vi "OutputSwerve.vi"() -> ()   [LabVIEW 2020]
doc: "This VI runs feedback and feedforward controllers, manages safety interlocks, and sends commands to the swerve drive and azimuth motors. This VI also controls the commanded drive shifter (low gear or high gear) state."
uses:
  744fb9e7-64fc-4bc7-b371-cd49665d8c00.vi
  bd7bff45-d105-4c72-b52f-b7d898b15bf8.vi
  e7293d0b-e8ab-4975-ac5b-493dfa430016.vi
  4db519e9-bae7-49f3-a1c3-53a7204bbb79.vi
  d610c66c-71b6-4d3a-a8b1-b399ee96c8a2.vi
  77f8b8d5-fd7b-4b62-a195-6ccd341d14a1.vi
  6abf8b40-ef0a-49e3-8d46-47362e9bd307.vi
  ae5b7493-7bbf-44c5-8d67-5f44d96a3e48.vi
  GlobalDriverStationData.vi
  GlobalDrivebase.vi
  TAI_Motor.vi
  GRNF_CTREMotor.vi
  GRNF_GenericSolenoid.vi
  TAI_Solenoid.vi
panel:
  in  "Azimuth PID Parameters":T1={"Kp"=0.3, "Ki"=0.0, "Kd"=0.0, "Kf (don't use)"=0.0, "I-Zone"=10.0} {"Kd" min=0.0; "Ki" min=0.0; "Kp" min=0.0}
  in  "Manual Azimuth Goal (deg) [-180,180]":dbl step=5.0
  in  "Manually Override Azimuth Goal":bool
  in  "Best Angle Hysteresis (deg)":dbl=20.0 format="%#_13g"
  out "Azimuth Position":cluster{dbl, "Interlock Output":dbl}(graph)
  out "Azimuth Error (deg)":dbl
  in  "Plotting":T2(ring)
  in  "Force to Low Gear":bool
  in  "Force To High Gear":bool
  in  "Drive Command Override [0,1]":dbl min=0.0 max=1.0 step=0.1
  in  "Manually Override Drive Command":bool
  in  "Time Below Speed (ms)":u32=150
  in  "Time Above Speed (ms)":u32=150
  in  "Switch to Low Gear (rpm)":dbl=500.0
  in  "Switch to High Gear (rpm)":dbl=3500.0
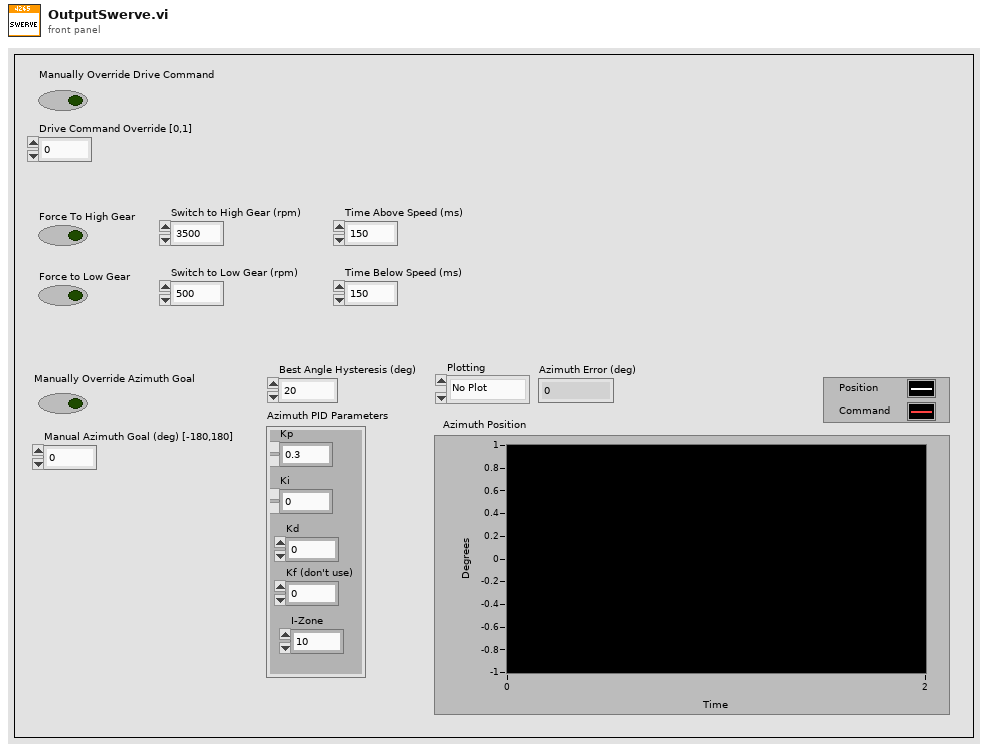
[diagram p1: front panel]
types:
  T1 = cluster{"Kp":dbl, "Ki":dbl, "Kd":dbl, "Kf (don't use)":dbl, "I-Zone":dbl}
  T2 = enum16{"No Plot", "Module 0", "Module 1", "Module 2", "Module 3"}
  T3 = enum16{"Safety", "Travelling", "Positioning", "Holding"}
  T4 = typedef "WPI_MotorControlDeviceRef.ctl" = cluster{"DeviceStatus":errorcluster, "Type":T5, "PWM":cluster{"PWM Channel":T6, "DeadBand":T7}, "CAN":cluster{"Device Number":u8, "SetOutput VI Ref":variant, "GetOutput VI Ref":variant, "Enable VI Ref":variant, "Disable VI Ref":variant, "Data":variant}, "Invert":bool, "DIO PWM":cluster{"PWM \"Enable\" Channel":T6, "DIOChannel":T8, "PWM Rate":dbl}}
  T5 = typedef "WPI_MotorControlType.ctl" = enum16{"PWM", "CAN", "DIO PWM"}
  T6 = typedef "FPGA_DIOPWMChannel.ctl" = enum8{"PWM 0", "PWM 1", "PWM 2", "PWM 3", "PWM 4", "PWM 5", "PWM 6", "PWM 7", "PWM 8", "PWM 9", "PWM MXP 0", "PWM MXP 1", "PWM MXP 2", "PWM MXP 3", "PWM MXP 4", "PWM MXP 5", "PWM MXP 6", "PWM MXP 7", "PWM MXP 8", "PWM MXP 9", "Invalid"}
  T7 = typedef "WPI_PWMDeadband.ctl" = cluster{"Name":string, "maxPositivePwm":i32, "minPositivePwm":i32, "centerPwm":i32, "maxNegativePwm":i32, "minNegativePwm":i32, "angularRange":u16}
  T8 = typedef "FPGA_DIOChannel.ctl" = enum8{"DIO 0", "DIO 1", "DIO 2", "DIO 3", "DIO 4", "DIO 5", "DIO 6", "DIO 7", "DIO 8", "DIO 9", "DIO MXP 0", "DIO MXP 1", "DIO MXP 2", "DIO MXP 3", "DIO MXP 4", "DIO MXP 5", "DIO MXP 6", "DIO MXP 7", "DIO MXP 8", "DIO MXP 9", "DIO MXP 10", "DIO MXP 11", "DIO MXP 12", "DIO MXP 13", "DIO MXP 14", "DIO MXP 15", "SPI Port CS1", "SPI Port CS2", "SPI Port CS3", "SPI Port MISO", "SPI Port MOSI", "Invalid"}
  T9 = enum16{"No Changed Output", "New Normal Output", "New Testing Output"}
  T10 = enum16{"Low Gear", "High Gear", "Transiting", "Unknown", "Force Low Gear"}
  T11 = cluster{"SEN_Azimuth_Position_Unwrapped_3 (deg)":dbl, dbl}
  T12 = typedef "WPI_SolenoidDevRef.ctl" = cluster{"DevStatus":errorcluster, "Pneumatics Control Module":u8, "Forward Solenoid Channel":T13, "Reverse Solenoid Channel":T13}
  T13 = typedef "WPI_SolenoidChannel.ctl" = enum8{"Solenoid 0", "Solenoid 1", "Solenoid 2", "Solenoid 3", "Solenoid 4", "Solenoid 5", "Solenoid 6", "Solenoid 7", "Solenoid 8", "Solenoid 9", "Solenoid 10", "Solenoid 11", "Solenoid 12", "Solenoid 13", "Solenoid 14", "Solenoid 15", "Invalid"}
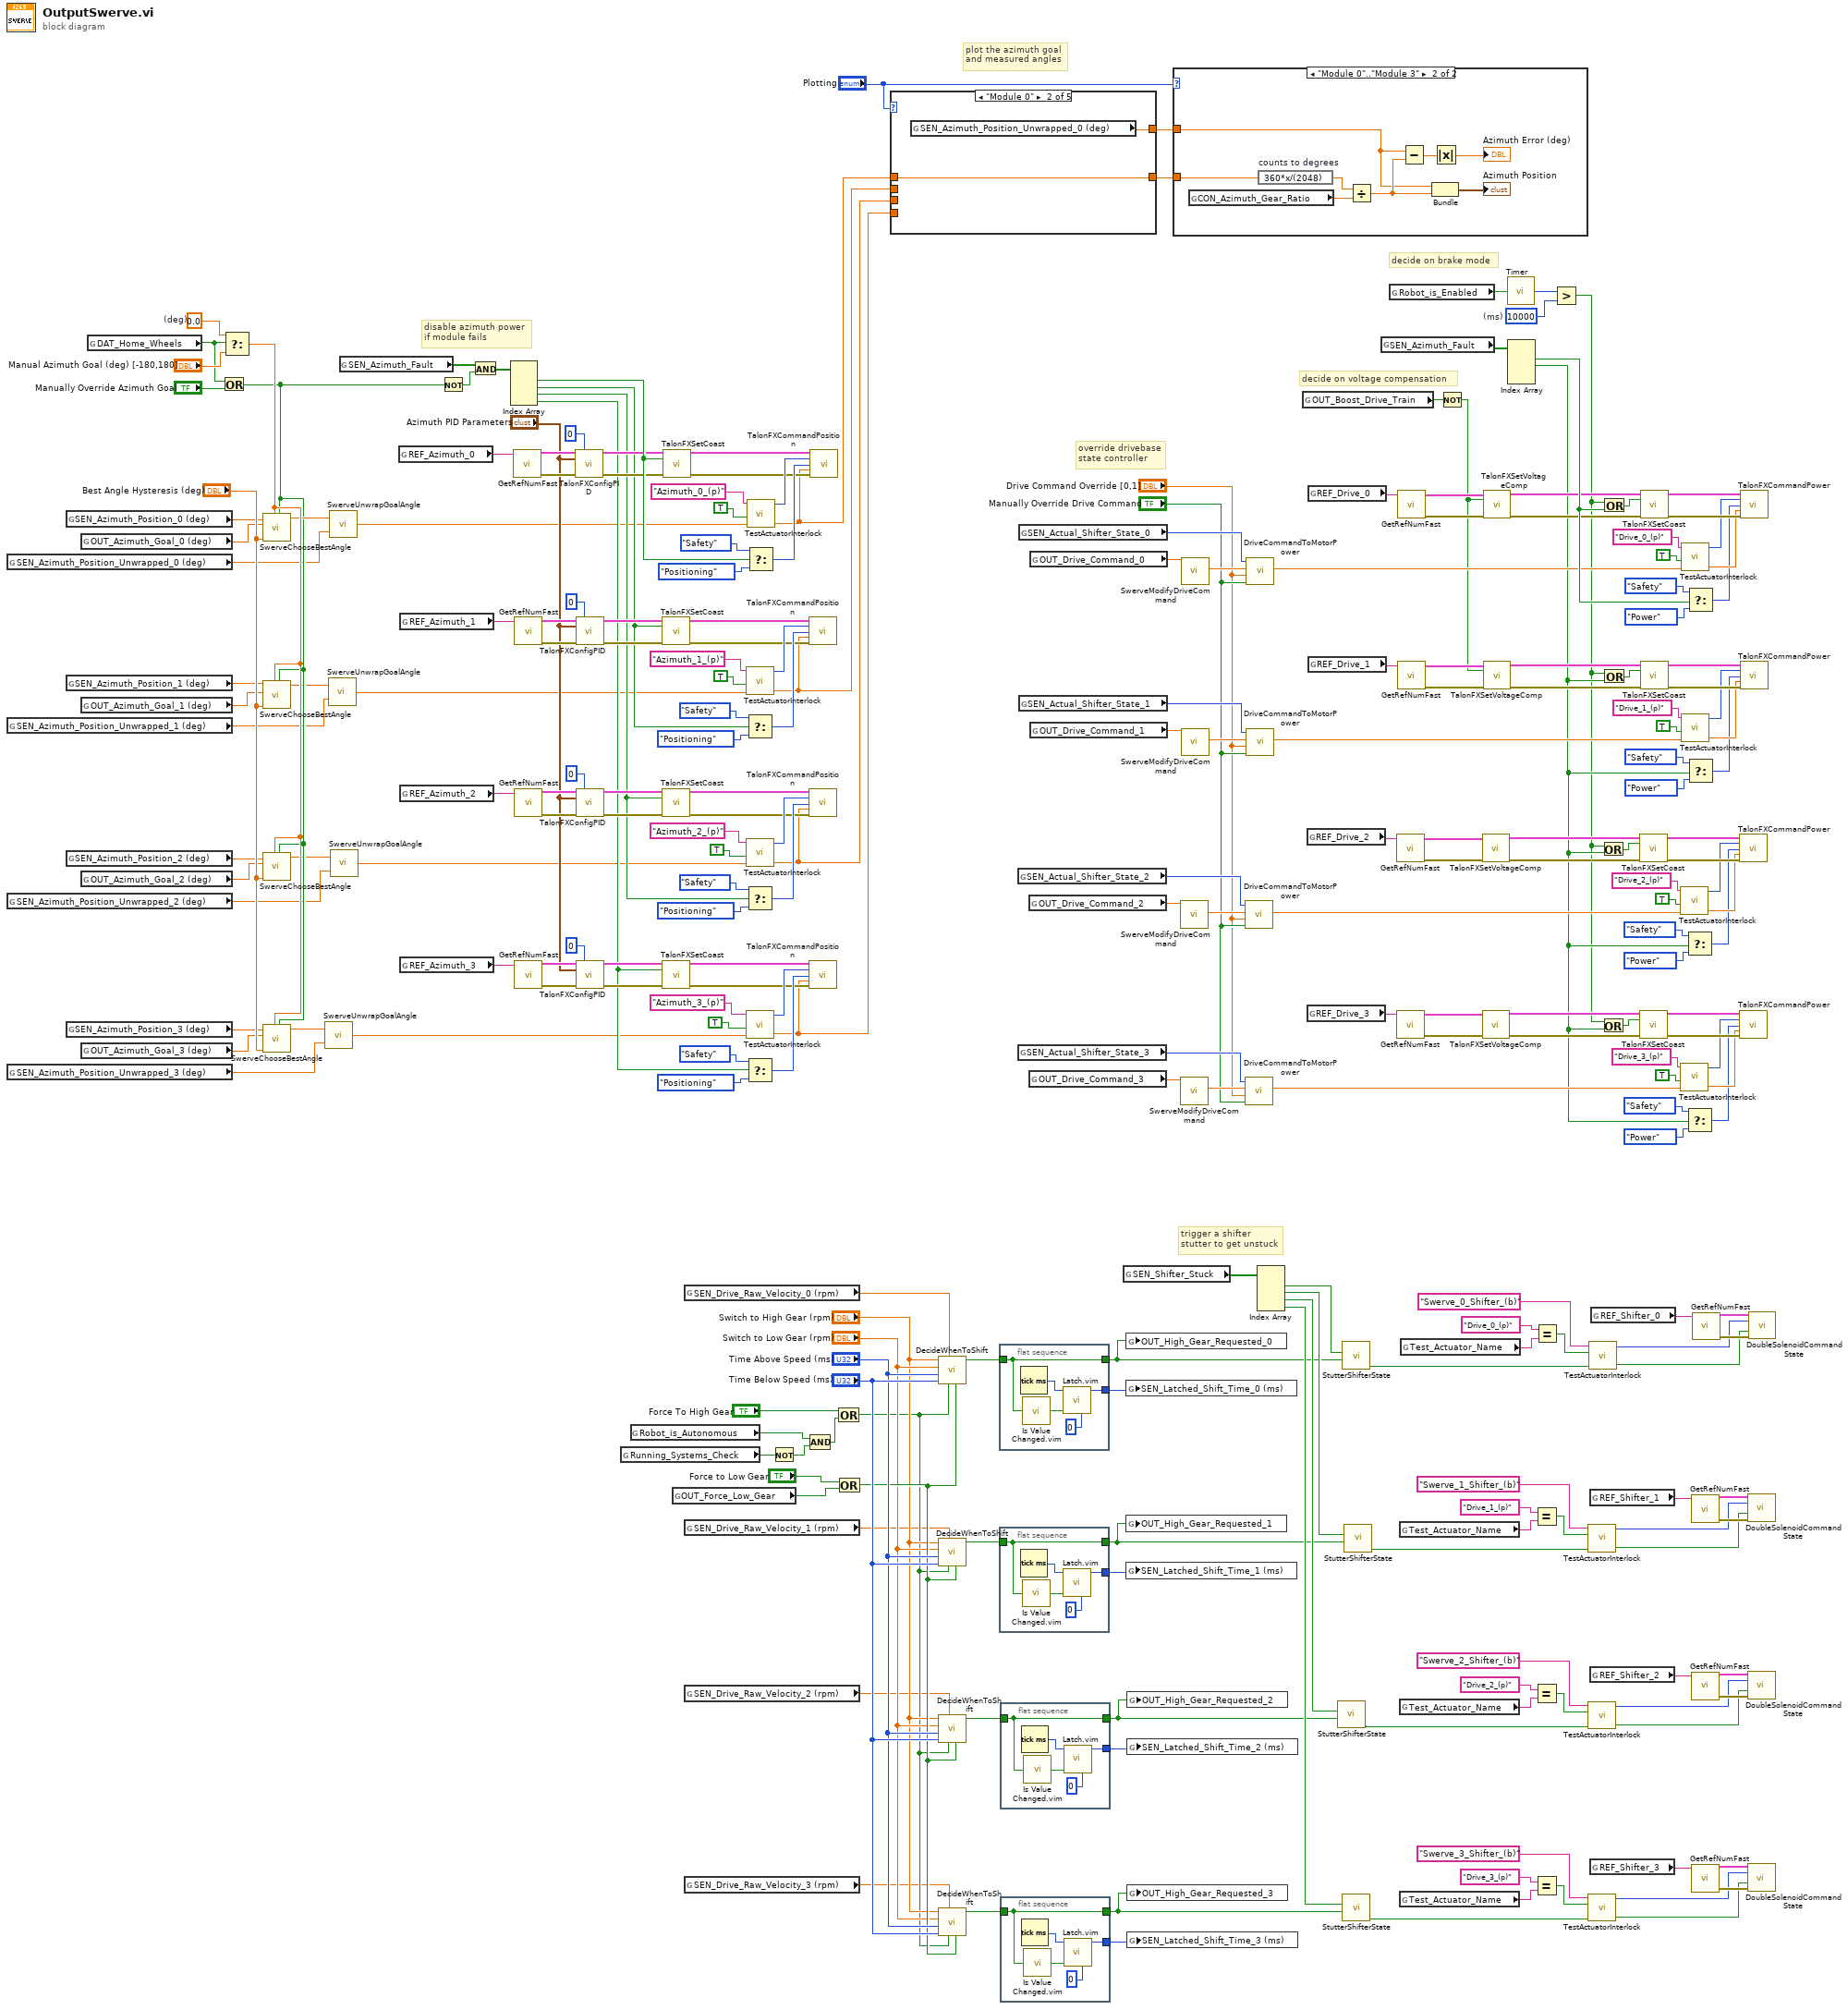
[diagram p0: block diagram]
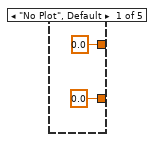
[diagram p3: hidden frame]
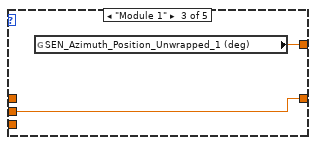
[diagram p4: hidden frame]
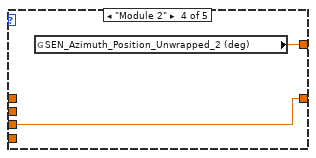
[diagram p5: hidden frame]
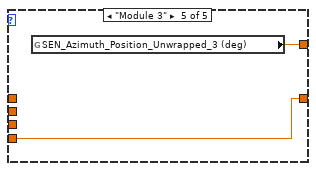
[diagram p6: hidden frame]
diagram:
  w97 = 0.0  # (deg)
  w230 = u32 10000  # (ms)
  # "plot the azimuth goal\nand measured angles"
  # "disable azimuth power\nif module fails"
  # "trigger a shifter\nstutter to get unstuck"
  # "override drivebase\nstate controller"
  # "decide on brake mode"
  # "decide on voltage compensation"
  n1 = global read "GlobalDrivebase.vi" "SEN_Azimuth_Position_Unwrapped_0 (deg)"() -> (w80:dbl)
  n2 = global read "GlobalDrivebase.vi" "SEN_Azimuth_Position_Unwrapped_1 (deg)"() -> (w78:dbl)
  n3 = global read "GlobalDrivebase.vi" "SEN_Azimuth_Position_Unwrapped_2 (deg)"() -> (w76:dbl)
  n4 = global read "GlobalDrivebase.vi" "SEN_Azimuth_Position_Unwrapped_3 (deg)"() -> (w74:dbl)
  n5 = global read "GlobalDrivebase.vi" "SEN_Azimuth_Position_0 (deg)"() -> (w81:dbl)
  n6 = global read "GlobalDrivebase.vi" "SEN_Azimuth_Position_1 (deg)"() -> (w79:dbl)
  n7 = global read "GlobalDrivebase.vi" "SEN_Azimuth_Position_2 (deg)"() -> (w77:dbl)
  n8 = global read "GlobalDrivebase.vi" "SEN_Azimuth_Position_3 (deg)"() -> (w75:dbl)
  n9 = global read "GlobalDrivebase.vi" "OUT_Azimuth_Goal_0 (deg)"() -> (w85:dbl)
  n10 = global read "GlobalDrivebase.vi" "OUT_Azimuth_Goal_1 (deg)"() -> (w84:dbl)
  n11 = global read "GlobalDrivebase.vi" "OUT_Azimuth_Goal_2 (deg)"() -> (w83:dbl)
  n12 = global read "GlobalDrivebase.vi" "OUT_Azimuth_Goal_3 (deg)"() -> (w82:dbl)
  n13 = global read "GlobalDrivebase.vi" "DAT_Home_Wheels"() -> (w10:bool)
  n14 = Or(x=w10, y="Manually Override Azimuth Goal") -> (x .or. y?=w90:bool)
  n15 = Select(t=w97, s=w10, f="Manual Azimuth Goal (deg) [-180,180]") -> (s? t:f=w96:dbl)
  n16 = call "SwerveChooseBestAngle.vi"("Goal Override"=w90, "Goal Override Angle (deg) [-180,+180]"=w96, "Hysteresis (deg)"="Best Angle Hysteresis (deg)", "Goal Angle (deg) [-180,+180]"=w85, "Current Angle (deg) [-180,+180]"=w81) -> ("Flipped Goal Angle (deg) [-180, +180]"=w94:dbl)  [unwired: 4 in, 2 out]
  n17 = call "SwerveChooseBestAngle.vi"("Goal Override"=w90, "Goal Override Angle (deg) [-180,+180]"=w96, "Hysteresis (deg)"="Best Angle Hysteresis (deg)", "Goal Angle (deg) [-180,+180]"=w84, "Current Angle (deg) [-180,+180]"=w79) -> ("Flipped Goal Angle (deg) [-180, +180]"=w88:dbl)  [unwired: 4 in, 2 out]
  n18 = call "SwerveChooseBestAngle.vi"("Goal Override"=w90, "Goal Override Angle (deg) [-180,+180]"=w96, "Hysteresis (deg)"="Best Angle Hysteresis (deg)", "Goal Angle (deg) [-180,+180]"=w83, "Current Angle (deg) [-180,+180]"=w77) -> ("Flipped Goal Angle (deg) [-180, +180]"=w87:dbl)  [unwired: 4 in, 2 out]
  n19 = call "SwerveChooseBestAngle.vi"("Goal Override"=w90, "Goal Override Angle (deg) [-180,+180]"=w96, "Hysteresis (deg)"="Best Angle Hysteresis (deg)", "Goal Angle (deg) [-180,+180]"=w82, "Current Angle (deg) [-180,+180]"=w75) -> ("Flipped Goal Angle (deg) [-180, +180]"=w86:dbl)  [unwired: 4 in, 2 out]
  n20 = call "SwerveUnwrapGoalAngle.vi"("Current Unwrapped Angle (deg) [-Inf,+Inf]"=w74, "Flipped Goal Angle (deg) [-180, +180]"=w86) -> ("Absolute Azimuth Position (tics) [-Inf,+Inf]"=w11:dbl)
  n21 = call "SwerveUnwrapGoalAngle.vi"("Current Unwrapped Angle (deg) [-Inf,+Inf]"=w78, "Flipped Goal Angle (deg) [-180, +180]"=w88) -> ("Absolute Azimuth Position (tics) [-Inf,+Inf]"=w13:dbl)
  n22 = call "SwerveUnwrapGoalAngle.vi"("Current Unwrapped Angle (deg) [-Inf,+Inf]"=w80, "Flipped Goal Angle (deg) [-180, +180]"=w94) -> ("Absolute Azimuth Position (tics) [-Inf,+Inf]"=w14:dbl)
  n23 = call "SwerveUnwrapGoalAngle.vi"("Current Unwrapped Angle (deg) [-Inf,+Inf]"=w76, "Flipped Goal Angle (deg) [-180, +180]"=w87) -> ("Absolute Azimuth Position (tics) [-Inf,+Inf]"=w12:dbl)
  n24 = global read "GlobalDrivebase.vi" "SEN_Azimuth_Fault"() -> (w73:bool[])
  n25 = global read "GlobalDrivebase.vi" "REF_Azimuth_0"() -> (w98:string)
  n26 = global read "GlobalDrivebase.vi" "REF_Azimuth_1"() -> (w59:string)
  n27 = global read "GlobalDrivebase.vi" "REF_Azimuth_2"() -> (w45:string)
  n28 = global read "GlobalDrivebase.vi" "REF_Azimuth_3"() -> (w29:string)
  n29 = Not(x=w90) -> (.not. x?=w91:bool)
  n30 = And(x=w73, y=w91) -> (x .and. y?=w92:bool[])
  n31 = Index Array(array=w92) -> (element #1=w66:bool, element #2=w47:bool, element #3=w33:bool, element #4=w15:bool)  [unwired: 4 in]
  n32 = call-poly "GetRefNumFast.vi"("RefNum Name"=w98) -> ("Error"=w62:errorcluster, "Device Reference"=w61:T4)  [unwired: 5 in]
  n33 = call-poly "GetRefNumFast.vi"("RefNum Name"=w59) -> ("Error"=w50:errorcluster, "Device Reference"=w49:T4)  [unwired: 5 in]
  n34 = call-poly "GetRefNumFast.vi"("RefNum Name"=w45) -> ("Error"=w36:errorcluster, "Device Reference"=w35:T4)  [unwired: 5 in]
  n35 = call-poly "GetRefNumFast.vi"("RefNum Name"=w29) -> ("Error"=w20:errorcluster, "Device Reference"=w19:T4)  [unwired: 5 in]
  n36 = call "TalonFXConfigPID.vi"("Device Reference (in)"=w61, "PID Slot"=0 ("slotIdx"), "PID Parameters"="Azimuth PID Parameters", "Error (in)"=w62) -> ("Device Reference (out)"=w64:T4, "Error (out)"=w63:errorcluster)  [unwired: 10 in]
  n37 = call "TalonFXConfigPID.vi"("Device Reference (in)"=w49, "PID Slot"=0 ("slotIdx"), "PID Parameters"="Azimuth PID Parameters", "Error (in)"=w50) -> ("Device Reference (out)"=w52:T4, "Error (out)"=w51:errorcluster)  [unwired: 10 in]
  n38 = call "TalonFXConfigPID.vi"("Device Reference (in)"=w35, "PID Slot"=0 ("slotIdx"), "PID Parameters"="Azimuth PID Parameters", "Error (in)"=w36) -> ("Device Reference (out)"=w38:T4, "Error (out)"=w37:errorcluster)  [unwired: 10 in]
  n39 = call "TalonFXConfigPID.vi"("Device Reference (in)"=w19, "PID Slot"=0 ("slotIdx"), "PID Parameters"="Azimuth PID Parameters", "Error (in)"=w20) -> ("Device Reference (out)"=w22:T4, "Error (out)"=w21:errorcluster)  [unwired: 10 in]
  n40 = global read "GlobalDriverStationData.vi" "Running_Systems_Check"() -> (w240:bool)
  n41 = global read "GlobalDriverStationData.vi" "Robot_is_Autonomous"() -> (w242:bool)
  n42 = call "TalonFXSetCoast.vi"("Device Reference (in)"=w52, "Set Coast Mode"=w47, "Error (in)"=w51) -> ("Device Reference (out)"=w6:T4, "Error (out)"=w53:errorcluster)  [unwired: 11 in]
  n43 = call "TalonFXSetCoast.vi"("Device Reference (in)"=w38, "Set Coast Mode"=w33, "Error (in)"=w37) -> ("Device Reference (out)"=w5:T4, "Error (out)"=w39:errorcluster)  [unwired: 11 in]
  n44 = call "TalonFXSetCoast.vi"("Device Reference (in)"=w22, "Set Coast Mode"=w15, "Error (in)"=w21) -> ("Device Reference (out)"=w4:T4, "Error (out)"=w23:errorcluster)  [unwired: 11 in]
  n45 = call "TalonFXSetCoast.vi"("Device Reference (in)"=w64, "Set Coast Mode"=w66, "Error (in)"=w63) -> ("Device Reference (out)"=w60:T4, "Error (out)"=w67:errorcluster)  [unwired: 11 in]
  n46 = global read "GlobalDrivebase.vi" "OUT_Force_Low_Gear"() -> (w237:bool)
  n47 = global read "GlobalDrivebase.vi" "SEN_Drive_Raw_Velocity_0 (rpm)"() -> (w102:dbl)
  n48 = global read "GlobalDrivebase.vi" "SEN_Drive_Raw_Velocity_1 (rpm)"() -> (w101:dbl)
  n49 = global read "GlobalDrivebase.vi" "SEN_Drive_Raw_Velocity_2 (rpm)"() -> (w100:dbl)
  n50 = global read "GlobalDrivebase.vi" "SEN_Drive_Raw_Velocity_3 (rpm)"() -> (w99:dbl)
  n51 = call-poly "TestActuatorInterlock.vi"("Normal Output"=w13, "Aux Trigger"=TRUE, "Actuator Name"="Azimuth_1_(p)" ("Actuator_Name")) -> ("Interlocked Output"=w46:dbl, "Output Mode"=w57:T9)  [unwired: 2 in]
  n52 = Select(t=T3."Safety" ("Control Mode"), s=w47, f=T3."Positioning") -> (s? t:f=w54:T3)
  n53 = call-poly "TestActuatorInterlock.vi"("Normal Output"=w12, "Aux Trigger"=TRUE, "Actuator Name"="Azimuth_2_(p)" ("Actuator_Name")) -> ("Interlocked Output"=w8:dbl, "Output Mode"=w43:T9)  [unwired: 2 in]
  n54 = Select(t=T3."Safety" ("Control Mode"), s=w33, f=T3."Positioning") -> (s? t:f=w40:T3)
  n55 = call-poly "TestActuatorInterlock.vi"("Normal Output"=w11, "Aux Trigger"=TRUE, "Actuator Name"="Azimuth_3_(p)" ("Actuator_Name")) -> ("Interlocked Output"=w7:dbl, "Output Mode"=w27:T9)  [unwired: 2 in]
  n56 = Select(t=T3."Safety" ("Control Mode"), s=w15, f=T3."Positioning") -> (s? t:f=w24:T3)
  n57 = call-poly "TestActuatorInterlock.vi"("Normal Output"=w14, "Aux Trigger"=TRUE, "Actuator Name"="Azimuth_0_(p)" ("Actuator_Name")) -> ("Interlocked Output"=w1:dbl, "Output Mode"=w71:T9)  [unwired: 2 in]
  n58 = Select(t=T3."Safety" ("Control Mode"), s=w66, f=T3."Positioning") -> (s? t:f=w68:T3)
  n59 = Not(x=w240) -> (.not. x?=w239:bool)
  n60 = call "TalonFXCommandPosition.vi"("Device Reference (in)"=w6, "Output Mode"=w57, "Control Mode"=w54, "Position (counts) or Testing Power"=w46, "Error (in)"=w53) -> ()  [unwired: 11 in]
  n61 = call "TalonFXCommandPosition.vi"("Device Reference (in)"=w5, "Output Mode"=w43, "Control Mode"=w40, "Position (counts) or Testing Power"=w8, "Error (in)"=w39) -> ()  [unwired: 11 in]
  n62 = call "TalonFXCommandPosition.vi"("Device Reference (in)"=w4, "Output Mode"=w27, "Control Mode"=w24, "Position (counts) or Testing Power"=w7, "Error (in)"=w23) -> ()  [unwired: 11 in]
  n63 = call "TalonFXCommandPosition.vi"("Device Reference (in)"=w60, "Output Mode"=w71, "Control Mode"=w68, "Position (counts) or Testing Power"=w1, "Error (in)"=w67) -> ()  [unwired: 11 in]
  n64 = Compound Arithmetic op=AND(w242, w239) -> (w241:bool)
  n65 = Compound Arithmetic op=OR("Force To High Gear", w241) -> (w243:bool)
  n66 = Compound Arithmetic op=OR("Force to Low Gear", w237) -> (w256:bool)
  n67 = case shown="\"Module 0\"" "Plotting" {
    tunnel: w1 -> [_ w263 _ _ _]
    tunnel: [0.0 ("Interlock Output") w263 w264 w267 w269] -> w93
    tunnel: w46 -> [_ _ w264 _ _]
    tunnel: w8 -> [_ _ _ w267 _]
    tunnel: w7 -> [_ _ _ _ w269]
    tunnel: [0.0 ("SEN_Azimuth_Position_Unwrapped_3 (deg)") w262 w265 w266 w268] -> w3
    frame "No Plot", Default {
    }
    frame "Module 0" {
      n68 = global read "GlobalDrivebase.vi" "SEN_Azimuth_Position_Unwrapped_0 (deg)"() -> (w262:dbl)
    }
    frame "Module 1" {
      n69 = global read "GlobalDrivebase.vi" "SEN_Azimuth_Position_Unwrapped_1 (deg)"() -> (w265:dbl)
    }
    frame "Module 2" {
      n70 = global read "GlobalDrivebase.vi" "SEN_Azimuth_Position_Unwrapped_2 (deg)"() -> (w266:dbl)
    }
    frame "Module 3" {
      n71 = global read "GlobalDrivebase.vi" "SEN_Azimuth_Position_Unwrapped_3 (deg)"() -> (w268:dbl)
    }
  }
  n72 = call "DecideWhenToShift.vi"("Force to Low Gear"=w256, "Force To High Gear"=w243, "Drive Motor Speed (rpm)"=w102, "Time Below Speed (ms)"="Time Below Speed (ms)", "Time Above Speed (ms)"="Time Above Speed (ms)", "Switch to Low Gear (rpm)"="Switch to Low Gear (rpm)", "Switch to High Gear (rpm)"="Switch to High Gear (rpm)") -> ("Requested Shifter State"=w251:bool)  [unwired: 4 in]
  n73 = call "DecideWhenToShift.vi"("Force to Low Gear"=w256, "Force To High Gear"=w243, "Drive Motor Speed (rpm)"=w101, "Time Below Speed (ms)"="Time Below Speed (ms)", "Time Above Speed (ms)"="Time Above Speed (ms)", "Switch to Low Gear (rpm)"="Switch to Low Gear (rpm)", "Switch to High Gear (rpm)"="Switch to High Gear (rpm)") -> ("Requested Shifter State"=w109:bool)  [unwired: 4 in]
  n74 = call "DecideWhenToShift.vi"("Force to Low Gear"=w256, "Force To High Gear"=w243, "Drive Motor Speed (rpm)"=w100, "Time Below Speed (ms)"="Time Below Speed (ms)", "Time Above Speed (ms)"="Time Above Speed (ms)", "Switch to Low Gear (rpm)"="Switch to Low Gear (rpm)", "Switch to High Gear (rpm)"="Switch to High Gear (rpm)") -> ("Requested Shifter State"=w107:bool)  [unwired: 4 in]
  n75 = call "DecideWhenToShift.vi"("Force to Low Gear"=w256, "Force To High Gear"=w243, "Drive Motor Speed (rpm)"=w99, "Time Below Speed (ms)"="Time Below Speed (ms)", "Time Above Speed (ms)"="Time Above Speed (ms)", "Switch to Low Gear (rpm)"="Switch to Low Gear (rpm)", "Switch to High Gear (rpm)"="Switch to High Gear (rpm)") -> ("Requested Shifter State"=w104:bool)  [unwired: 4 in]
  n76 = flat-sequence {
    tunnel: w251 -> [w272]
    tunnel: [w272] -> w113
    tunnel: [w270] -> w112
    frame #0 {
      n77 = Tick Count (ms)() -> (millisecond timer value=w274:u32)
      n78 = call "Is Value Changed.vim"("value"=w272) -> ("changed or first call?"=w271:bool)
      n79 = call "Latch.vim"("Default Value"=u32 0 ("millisecond timer value"), "Latch Signal"=w271, "Latch Value"=w274) -> ("Latched"=w270:u32)  [unwired: 8 in]
    }
  }
  n80 = flat-sequence {
    tunnel: w109 -> [w277]
    tunnel: [w277] -> w110
    tunnel: [w275] -> w111
    frame #0 {
      n81 = Tick Count (ms)() -> (millisecond timer value=w279:u32)
      n82 = call "Is Value Changed.vim"("value"=w277) -> ("changed or first call?"=w276:bool)
      n83 = call "Latch.vim"("Default Value"=u32 0 ("millisecond timer value"), "Latch Signal"=w276, "Latch Value"=w279) -> ("Latched"=w275:u32)  [unwired: 8 in]
    }
  }
  n84 = flat-sequence {
    tunnel: w107 -> [w282]
    tunnel: [w282] -> w106
    tunnel: [w280] -> w108
    frame #0 {
      n85 = Tick Count (ms)() -> (millisecond timer value=w284:u32)
      n86 = call "Is Value Changed.vim"("value"=w282) -> ("changed or first call?"=w281:bool)
      n87 = call "Latch.vim"("Default Value"=u32 0 ("millisecond timer value"), "Latch Signal"=w281, "Latch Value"=w284) -> ("Latched"=w280:u32)  [unwired: 8 in]
    }
  }
  n88 = flat-sequence {
    tunnel: w104 -> [w287]
    tunnel: [w287] -> w103
    tunnel: [w285] -> w105
    frame #0 {
      n89 = Tick Count (ms)() -> (millisecond timer value=w289:u32)
      n90 = call "Is Value Changed.vim"("value"=w287) -> ("changed or first call?"=w286:bool)
      n91 = call "Latch.vim"("Default Value"=u32 0 ("millisecond timer value"), "Latch Signal"=w286, "Latch Value"=w289) -> ("Latched"=w285:u32)  [unwired: 8 in]
    }
  }
  n92 = global read "GlobalDrivebase.vi" "SEN_Actual_Shifter_State_2"() -> (w190:T10)
  n93 = global read "GlobalDrivebase.vi" "SEN_Actual_Shifter_State_3"() -> (w171:T10)
  n94 = global read "GlobalDrivebase.vi" "SEN_Actual_Shifter_State_0"() -> (w236:T10)
  n95 = global read "GlobalDrivebase.vi" "SEN_Actual_Shifter_State_1"() -> (w210:T10)
  n96 = global read "GlobalDrivebase.vi" "OUT_Drive_Command_2"() -> (w191:dbl)
  n97 = global read "GlobalDrivebase.vi" "OUT_Drive_Command_3"() -> (w172:dbl)
  n98 = global read "GlobalDrivebase.vi" "OUT_Drive_Command_0"() -> (w238:dbl)
  n99 = global read "GlobalDrivebase.vi" "OUT_Drive_Command_1"() -> (w211:dbl)
  n100 = global read "GlobalDrivebase.vi" "SEN_Shifter_Stuck"() -> (w235:bool[])
  n101 = global write "GlobalDrivebase.vi" "OUT_High_Gear_Requested_0"(w113) -> ()
  n102 = global write "GlobalDrivebase.vi" "SEN_Latched_Shift_Time_0 (ms)"(w112) -> ()
  n103 = global write "GlobalDrivebase.vi" "OUT_High_Gear_Requested_1"(w110) -> ()
  n104 = global write "GlobalDrivebase.vi" "SEN_Latched_Shift_Time_1 (ms)"(w111) -> ()
  n105 = global write "GlobalDrivebase.vi" "OUT_High_Gear_Requested_2"(w106) -> ()
  n106 = global write "GlobalDrivebase.vi" "SEN_Latched_Shift_Time_2 (ms)"(w108) -> ()
  n107 = global write "GlobalDrivebase.vi" "OUT_High_Gear_Requested_3"(w103) -> ()
  n108 = global write "GlobalDrivebase.vi" "SEN_Latched_Shift_Time_3 (ms)"(w105) -> ()
  n109 = case shown="\"Module 0\"..\"Module 3\"" "Plotting" {
    tunnel: w93 -> [_ w296]
    tunnel: w3 -> [_ w290]
    frame "No Plot", Default {
    }
    frame "Module 0".."Module 3" {
      n110 = global read "GlobalDrivebase.vi" "CON_Azimuth_Gear_Ratio"() -> (w291:dbl)
      n111 = expression code="360*x/(2048)" "counts to degrees"(w296) -> (w293:dbl)
      n112 = Divide(x=w293, y=w291) -> (x/y=w292:dbl)
      n113 = Subtract(x=w290, y=w292) -> (x-y=w295:dbl)
      n114 = Bundle("SEN_Azimuth_Position_Unwrapped_3 (deg)"=w290, w292) -> (→"Azimuth Position":T11)  [unwired: 1 in]
      n115 = Absolute Value(x=w295) -> (abs(x)=→"Azimuth Error (deg)":dbl)
    }
  }
  n116 = call "SwerveModifyDriveCommand.vi"("Raw Drive Command (ul)"=w191) -> ("Modified Drive Command (ul)"=w173:dbl)  [unwired: 5 in]
  n117 = call "SwerveModifyDriveCommand.vi"("Raw Drive Command (ul)"=w172) -> ("Modified Drive Command (ul)"=w154:dbl)  [unwired: 5 in]
  n118 = call "SwerveModifyDriveCommand.vi"("Raw Drive Command (ul)"=w238) -> ("Modified Drive Command (ul)"=w212:dbl)  [unwired: 5 in]
  n119 = call "SwerveModifyDriveCommand.vi"("Raw Drive Command (ul)"=w211) -> ("Modified Drive Command (ul)"=w193:dbl)  [unwired: 5 in]
  n120 = call "DriveCommandToMotorPower.vi"("Drive Command Override"="Manually Override Drive Command", "Drive Command Override (ul) [-1,1]"="Drive Command Override [0,1]", "Drive Command (ul) [-1,1]"=w173, "Actual Shifter State"=w190) -> ("Motor Power (ul) [-1,1]"=w174:dbl)  [unwired: 7 in]
  n121 = call "DriveCommandToMotorPower.vi"("Drive Command Override"="Manually Override Drive Command", "Drive Command Override (ul) [-1,1]"="Drive Command Override [0,1]", "Drive Command (ul) [-1,1]"=w154, "Actual Shifter State"=w171) -> ("Motor Power (ul) [-1,1]"=w155:dbl)  [unwired: 7 in]
  n122 = call "DriveCommandToMotorPower.vi"("Drive Command Override"="Manually Override Drive Command", "Drive Command Override (ul) [-1,1]"="Drive Command Override [0,1]", "Drive Command (ul) [-1,1]"=w212, "Actual Shifter State"=w236) -> ("Motor Power (ul) [-1,1]"=w213:dbl)  [unwired: 7 in]
  n123 = call "DriveCommandToMotorPower.vi"("Drive Command Override"="Manually Override Drive Command", "Drive Command Override (ul) [-1,1]"="Drive Command Override [0,1]", "Drive Command (ul) [-1,1]"=w193, "Actual Shifter State"=w210) -> ("Motor Power (ul) [-1,1]"=w194:dbl)  [unwired: 7 in]
  n124 = Index Array(array=w235) -> (element #1=w255:bool, element #2=w254:bool, element #3=w253:bool, element #4=w252:bool)  [unwired: 4 in]
  n125 = global read "GlobalDrivebase.vi" "OUT_Boost_Drive_Train"() -> (w214:bool)
  n126 = global read "GlobalDrivebase.vi" "REF_Drive_2"() -> (w188:string)
  n127 = global read "GlobalDrivebase.vi" "REF_Drive_3"() -> (w169:string)
  n128 = global read "GlobalDrivebase.vi" "REF_Drive_0"() -> (w233:string)
  n129 = global read "GlobalDrivebase.vi" "REF_Drive_1"() -> (w208:string)
  n130 = call "StutterShifterState.vi"("Requested Shifter State"=w106, "Request Stutter"=w253) -> ("Stuttered Shifter State"=w124:bool)  [unwired: 9 in]
  n131 = call "StutterShifterState.vi"("Requested Shifter State"=w113, "Request Stutter"=w255) -> ("Stuttered Shifter State"=w134:bool)  [unwired: 9 in]
  n132 = call "StutterShifterState.vi"("Requested Shifter State"=w103, "Request Stutter"=w252) -> ("Stuttered Shifter State"=w114:bool)  [unwired: 9 in]
  n133 = call "StutterShifterState.vi"("Requested Shifter State"=w110, "Request Stutter"=w254) -> ("Stuttered Shifter State"=w135:bool)  [unwired: 9 in]
  n134 = global read "GlobalDrivebase.vi" "SEN_Azimuth_Fault"() -> (w229:bool[])
  n135 = global read "GlobalDriverStationData.vi" "Robot_is_Enabled"() -> (w228:bool)
  n136 = call-poly "GetRefNumFast.vi"("RefNum Name"=w188) -> ("Error"=w177:errorcluster, "Device Reference"=w178:T4)  [unwired: 5 in]
  n137 = call-poly "GetRefNumFast.vi"("RefNum Name"=w169) -> ("Error"=w158:errorcluster, "Device Reference"=w159:T4)  [unwired: 5 in]
  n138 = call-poly "GetRefNumFast.vi"("RefNum Name"=w233) -> ("Error"=w217:errorcluster, "Device Reference"=w218:T4)  [unwired: 5 in]
  n139 = call-poly "GetRefNumFast.vi"("RefNum Name"=w208) -> ("Error"=w197:errorcluster, "Device Reference"=w198:T4)  [unwired: 5 in]
  n140 = global read "GlobalDriverStationData.vi" "Test_Actuator_Name"() -> (w142:string)
  n141 = global read "GlobalDriverStationData.vi" "Test_Actuator_Name"() -> (w131:string)
  n142 = global read "GlobalDriverStationData.vi" "Test_Actuator_Name"() -> (w121:string)
  n143 = global read "GlobalDriverStationData.vi" "Test_Actuator_Name"() -> (w247:string)
  n144 = Not(x=w214) -> (.not. x?=w192:bool)
  n145 = call "TalonFXSetVoltageComp.vi"("Device Reference (in)"=w178, "Error (in)"=w177) -> ("Device Reference (out)"=w176:T4, "Error (out)"=w175:errorcluster)  [unwired: 12 in]
  n146 = call "TalonFXSetVoltageComp.vi"("Device Reference (in)"=w159, "Error (in)"=w158) -> ("Device Reference (out)"=w157:T4, "Error (out)"=w156:errorcluster)  [unwired: 12 in]
  n147 = call "TalonFXSetVoltageComp.vi"("Device Reference (in)"=w218, "Set Voltage Compensation Mode"=w192, "Error (in)"=w217) -> ("Device Reference (out)"=w216:T4, "Error (out)"=w215:errorcluster)  [unwired: 11 in]
  n148 = call "TalonFXSetVoltageComp.vi"("Device Reference (in)"=w198, "Set Voltage Compensation Mode"=w192, "Error (in)"=w197) -> ("Device Reference (out)"=w196:T4, "Error (out)"=w195:errorcluster)  [unwired: 11 in]
  n149 = call "Timer.vi"("Reset Timer"=w228) -> ("Time (ms)"=w231:u32)
  n150 = Index Array(array=w229) -> (element #1=w219:bool, element #2=w151:bool)  [unwired: 4 in, 2 out]
  n151 = Equal?(x="Drive_1_(p)" ("Actuator_Name"), y=w142) -> (x = y?=w141:bool)
  n152 = Equal?(x="Drive_2_(p)" ("Actuator_Name"), y=w131) -> (x = y?=w130:bool)
  n153 = Equal?(x="Drive_3_(p)" ("Actuator_Name"), y=w121) -> (x = y?=w120:bool)
  n154 = Equal?(x="Drive_0_(p)" ("Actuator_Name"), y=w247) -> (x = y?=w246:bool)
  n155 = Greater?(x=w231, y=w230) -> (0:w150:bool)
  n156 = call-poly "TestActuatorInterlock.vi"("Normal Output"=w135, "Override Actuator Bypass"=w141, "Actuator Name"="Swerve_1_Shifter_(b)" ("Actuator_Name")) -> ("Interlocked Output"=w136:bool, "Output Mode"=w137:T9)  [unwired: 2 in]
  n157 = call-poly "TestActuatorInterlock.vi"("Normal Output"=w124, "Override Actuator Bypass"=w130, "Actuator Name"="Swerve_2_Shifter_(b)" ("Actuator_Name")) -> ("Interlocked Output"=w125:bool, "Output Mode"=w126:T9)  [unwired: 2 in]
  n158 = call-poly "TestActuatorInterlock.vi"("Normal Output"=w114, "Override Actuator Bypass"=w120, "Actuator Name"="Swerve_3_Shifter_(b)" ("Actuator_Name")) -> ("Interlocked Output"=w115:bool, "Output Mode"=w116:T9)  [unwired: 2 in]
  n159 = call-poly "TestActuatorInterlock.vi"("Normal Output"=w134, "Override Actuator Bypass"=w246, "Actuator Name"="Swerve_0_Shifter_(b)" ("Actuator_Name")) -> ("Interlocked Output"=w145:bool, "Output Mode"=w146:T9)  [unwired: 2 in]
  n160 = global read "GlobalDrivebase.vi" "REF_Shifter_1"() -> (w140:string)
  n161 = global read "GlobalDrivebase.vi" "REF_Shifter_2"() -> (w129:string)
  n162 = global read "GlobalDrivebase.vi" "REF_Shifter_3"() -> (w119:string)
  n163 = global read "GlobalDrivebase.vi" "REF_Shifter_0"() -> (w149:string)
  n164 = Or(x=w150, y=w151) -> (x .or. y?=w187:bool)
  n165 = Or(x=w150, y=w151) -> (x .or. y?=w168:bool)
  n166 = Or(x=w150, y=w219) -> (x .or. y?=w232:bool)
  n167 = Or(x=w150, y=w151) -> (x .or. y?=w207:bool)
  n168 = call "TalonFXSetCoast.vi"("Device Reference (in)"=w176, "Set Coast Mode"=w187, "Error (in)"=w175) -> ("Device Reference (out)"=w185:T4, "Error (out)"=w184:errorcluster)  [unwired: 11 in]
  n169 = call "TalonFXSetCoast.vi"("Device Reference (in)"=w157, "Set Coast Mode"=w168, "Error (in)"=w156) -> ("Device Reference (out)"=w166:T4, "Error (out)"=w165:errorcluster)  [unwired: 11 in]
  n170 = call "TalonFXSetCoast.vi"("Device Reference (in)"=w216, "Set Coast Mode"=w232, "Error (in)"=w215) -> ("Device Reference (out)"=w226:T4, "Error (out)"=w225:errorcluster)  [unwired: 11 in]
  n171 = call "TalonFXSetCoast.vi"("Device Reference (in)"=w196, "Set Coast Mode"=w207, "Error (in)"=w195) -> ("Device Reference (out)"=w205:T4, "Error (out)"=w204:errorcluster)  [unwired: 11 in]
  n172 = call-poly "TestActuatorInterlock.vi"("Normal Output"=w174, "Aux Trigger"=TRUE, "Actuator Name"="Drive_2_(p)" ("Actuator_Name")) -> ("Interlocked Output"=w183:dbl, "Output Mode"=w182:T9)  [unwired: 2 in]
  n173 = call-poly "TestActuatorInterlock.vi"("Normal Output"=w155, "Aux Trigger"=TRUE, "Actuator Name"="Drive_3_(p)" ("Actuator_Name")) -> ("Interlocked Output"=w164:dbl, "Output Mode"=w163:T9)  [unwired: 2 in]
  n174 = call-poly "TestActuatorInterlock.vi"("Normal Output"=w213, "Aux Trigger"=TRUE, "Actuator Name"="Drive_0_(p)" ("Actuator_Name")) -> ("Interlocked Output"=w224:dbl, "Output Mode"=w223:T9)  [unwired: 2 in]
  n175 = call-poly "TestActuatorInterlock.vi"("Normal Output"=w194, "Aux Trigger"=TRUE, "Actuator Name"="Drive_1_(p)" ("Actuator_Name")) -> ("Interlocked Output"=w203:dbl, "Output Mode"=w202:T9)  [unwired: 2 in]
  n176 = Select(t=enum16{"Safety", "Power"}."Safety" ("Control Mode"), s=w151, f=enum16{"Safety", "Power"}."Power") -> (s? t:f=w180:enum16{"Safety", "Power"})
  n177 = Select(t=enum16{"Safety", "Power"}."Safety" ("Control Mode"), s=w151, f=enum16{"Safety", "Power"}."Power") -> (s? t:f=w161:enum16{"Safety", "Power"})
  n178 = Select(t=enum16{"Safety", "Power"}."Safety" ("Control Mode"), s=w219, f=enum16{"Safety", "Power"}."Power") -> (s? t:f=w221:enum16{"Safety", "Power"})
  n179 = Select(t=enum16{"Safety", "Power"}."Safety" ("Control Mode"), s=w151, f=enum16{"Safety", "Power"}."Power") -> (s? t:f=w200:enum16{"Safety", "Power"})
  n180 = call-poly "GetRefNumFast.vi"("RefNum Name"=w140) -> ("Error"=w138:errorcluster, "Device Reference"=w139:T12)  [unwired: 5 in]
  n181 = call-poly "GetRefNumFast.vi"("RefNum Name"=w129) -> ("Error"=w127:errorcluster, "Device Reference"=w128:T12)  [unwired: 5 in]
  n182 = call-poly "GetRefNumFast.vi"("RefNum Name"=w119) -> ("Error"=w117:errorcluster, "Device Reference"=w118:T12)  [unwired: 5 in]
  n183 = call-poly "GetRefNumFast.vi"("RefNum Name"=w149) -> ("Error"=w147:errorcluster, "Device Reference"=w148:T12)  [unwired: 5 in]
  n184 = call "TalonFXCommandPower.vi"("Device Reference (in)"=w185, "Output Mode"=w182, "Control Mode"=w180, "Power or Testing Power"=w183, "Error (in)"=w184) -> ()  [unwired: 11 in]
  n185 = call "TalonFXCommandPower.vi"("Device Reference (in)"=w166, "Output Mode"=w163, "Control Mode"=w161, "Power or Testing Power"=w164, "Error (in)"=w165) -> ()  [unwired: 11 in]
  n186 = call "TalonFXCommandPower.vi"("Device Reference (in)"=w226, "Output Mode"=w223, "Control Mode"=w221, "Power or Testing Power"=w224, "Error (in)"=w225) -> ()  [unwired: 11 in]
  n187 = call "TalonFXCommandPower.vi"("Device Reference (in)"=w205, "Output Mode"=w202, "Control Mode"=w200, "Power or Testing Power"=w203, "Error (in)"=w204) -> ()  [unwired: 11 in]
  n188 = call "DoubleSolenoidCommandState.vi"("Device Reference (in)"=w139, "Output Mode"=w137, "State [True, False]"=w136, "Error (in)"=w138) -> ()  [unwired: 12 in]
  n189 = call "DoubleSolenoidCommandState.vi"("Device Reference (in)"=w128, "Output Mode"=w126, "State [True, False]"=w125, "Error (in)"=w127) -> ()  [unwired: 12 in]
  n190 = call "DoubleSolenoidCommandState.vi"("Device Reference (in)"=w118, "Output Mode"=w116, "State [True, False]"=w115, "Error (in)"=w117) -> ()  [unwired: 12 in]
  n191 = call "DoubleSolenoidCommandState.vi"("Device Reference (in)"=w148, "Output Mode"=w146, "State [True, False]"=w145, "Error (in)"=w147) -> ()  [unwired: 12 in]
